vi "Get Image Format.vi"(8 "错误输入（无错误）":errorcluster, 11 "Output Image Type":T1(ring)) -> (0 "错误输出":errorcluster, 3 "Image Format":refnum<k24>)   [LabVIEW 2011, in "Image Converter.lvlib"]
uses:
  Image Converter.lvlib
  System.Drawing
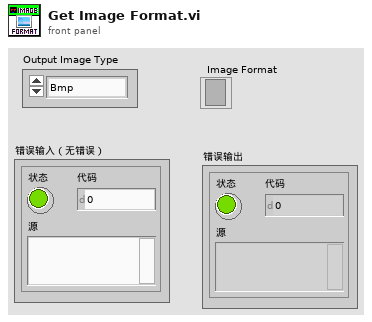
[diagram p1: front panel]
types:
  T1 = enum16{"Bmp", "Emf", "Exif", "Gif", "Icon", "Jpeg", "MemoryBmp", "Png", "Tiff", "Wmf"}
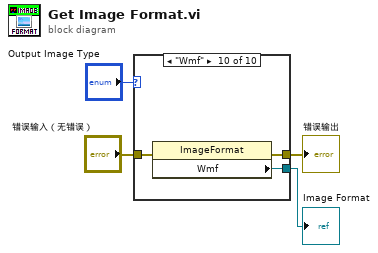
[diagram p0: block diagram]
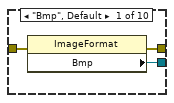
[diagram p2: hidden frame]
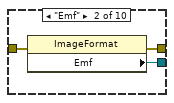
[diagram p3: hidden frame]
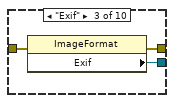
[diagram p4: hidden frame]
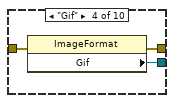
[diagram p5: hidden frame]
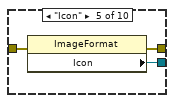
[diagram p6: hidden frame]
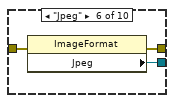
[diagram p7: hidden frame]
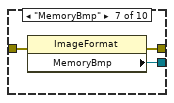
[diagram p8: hidden frame]
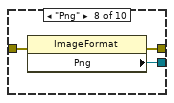
[diagram p9: hidden frame]
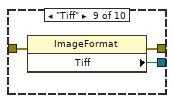
[diagram p10: hidden frame]
diagram:
  n1 = case shown="\"Wmf\"" "Output Image Type" {
    tunnel: [w7 w10 w13 w15 w18 w21 w24 w28 w31 w34] -> w3
    tunnel: [w5 w9 w12 w16 w19 w22 w25 w27 w30 w33] -> w1
    tunnel: "错误输入（无错误）" -> [w6 w8 w11 w14 w17 w20 w23 w26 w29 w32]
    frame "Bmp", Default {
      n2 = property class="ImageFormat"(error in=w6) -> (error out=w5:errorcluster, "Bmp"=w7:refnum<k24>)  [unwired: 1 in, 1 out]
    }
    frame "Emf" {
      n3 = property class="ImageFormat"(error in=w8) -> (error out=w9:errorcluster, "Emf"=w10:refnum<k24>)  [unwired: 1 in, 1 out]
    }
    frame "Exif" {
      n4 = property class="ImageFormat"(error in=w11) -> (error out=w12:errorcluster, "Exif"=w13:refnum<k24>)  [unwired: 1 in, 1 out]
    }
    frame "Gif" {
      n5 = property class="ImageFormat"(error in=w14) -> (error out=w16:errorcluster, "Gif"=w15:refnum<k24>)  [unwired: 1 in, 1 out]
    }
    frame "Icon" {
      n6 = property class="ImageFormat"(error in=w17) -> (error out=w19:errorcluster, "Icon"=w18:refnum<k24>)  [unwired: 1 in, 1 out]
    }
    frame "Jpeg" {
      n7 = property class="ImageFormat"(error in=w20) -> (error out=w22:errorcluster, "Jpeg"=w21:refnum<k24>)  [unwired: 1 in, 1 out]
    }
    frame "MemoryBmp" {
      n8 = property class="ImageFormat"(error in=w23) -> (error out=w25:errorcluster, "MemoryBmp"=w24:refnum<k24>)  [unwired: 1 in, 1 out]
    }
    frame "Png" {
      n9 = property class="ImageFormat"(error in=w26) -> (error out=w27:errorcluster, "Png"=w28:refnum<k24>)  [unwired: 1 in, 1 out]
    }
    frame "Tiff" {
      n10 = property class="ImageFormat"(error in=w29) -> (error out=w30:errorcluster, "Tiff"=w31:refnum<k24>)  [unwired: 1 in, 1 out]
    }
    frame "Wmf" {
      n11 = property class="ImageFormat"(error in=w32) -> (error out=w33:errorcluster, "Wmf"=w34:refnum<k24>)  [unwired: 1 in, 1 out]
    }
  }
  "Image Format" <- w3
  "错误输出" <- w1
